vi "Calibration pFC Data.vi"() -> ()   [LabVIEW 2014]
uses:
  <vilib>/Utility/file.llb/Read From Spreadsheet File (DBL).vi
  <vilib>/gmath/NumericalOptimization/Nonlinear Curve Fit LM formula string.vi
  <vilib>/Utility/file.llb/Write To Spreadsheet File (DBL).vi
  <vilib>/Analysis/NI_AALBase.lvlib
  <vilib>/gmath/NI_Gmath.lvlib
  <vilib>/Analysis/NI_AALPro.lvlib
panel:
  out "Selected xDNA (m51 count)":dbl[](array[numeric])
  out "Selected filt xDNA (m51 count)":dbl[](array[numeric])
  out "Selected xDNA (nm)":dbl[](array[numeric])
  in  "Final cut (s)":dbl=120.0
  out "Force (pN)":dbl
  out "read file path":path
  out "Fraction (f-u)":dbl[](array[numeric])
  out "Funfold (%)":dbl
  out "Ffold (%)":dbl
  out "path":path
  in  "Fit?":bool
  in  "initial parameters":dbl[](array[numeric])=[200.0, 1100.0, 6.0, 500.0, 1120.0, 6.0]
  out "Laser Power (mV)":dbl
  out "Data rate (Hz)":dbl
  in  "Tab Control 2":enum32{"Folder", "File"}(tab)
  in  "Folder Path":path
  in  "file path (dialog if empty)":path
  in  "intervals for selected xDNA":i32=100
  out "Histogram: h(x)":i32[](array[numeric])
  out "Selected filt xDNA (nm)":dbl[](array[numeric])
  out "Selected Time (s)":dbl[](array[numeric]) format="%_7g"
  in  "Selected tf (s)":dbl=10.0
  in  "Selected ti (s)":dbl
  out "Time for total (s)":dbl[](array[numeric])
  out "Total Filtered xDNA (nm)":dbl[](array[numeric])
  out "Data rate for total (Hz)":dbl
  in  "Filter for total":T1(ring)=enum."Moving-window avg"
  in  "#Avg for total":i32=5
  in  "# of adjencent points":i32=5
  in  "Save?":bool
  out "Target QPD (V)":dbl
  out "Total xDNA (nm)":dbl[](array[numeric])
  in  "Filter for initial":T1(ring)
  out "Total Peak location (index)":i32[](array[numeric])
  out "Each first and end diff":dbl[](array[numeric])
  out "Total xDNA":dbl[][](array[numeric])
  out "cut-xDNA (nm)":dbl[](array[numeric])
  out "xDNA diff (i-(i+1))":dbl[](array[numeric])
  out "New stage moved index":i32[](array[numeric])
  in  "initial cut (s)":dbl=0.1
  out "Stage moved time index":i32[](array[numeric])
  out "Stage moved time (s)":dbl[](array[numeric])
  out "Time Array (s)":dbl[](array[numeric])
  out "xDNA (nm)":dbl[](array[numeric])
  in  "Tab Control":T2(tab)
  out "XY Graph 4":cluster{dbl[], "Filtered QPD data":dbl[]}[](graph)
  out "XY Graph":cluster{dbl[], dbl[]}(graph)
  out "Each first and end":dbl[](array[numeric])
  out "Each Section First and End index":i32[](array[numeric])
  out "XY Graph 2":cluster{dbl[], dbl[]}(graph)
  out "Waveform Graph":dbl[][](graph)
  out "XY Graph 3":cluster{dbl[], "Filtered QPD data":dbl[]}[](graph)
  out "XY Graph 8":cluster{"power":dbl[], "Slope":dbl[]}(graph)
  out "XY Graph 5":cluster{dbl[], dbl[]}[](graph)
  out "Histogram Graph":T3(graph)
  out "best fit parameters":dbl[](array[numeric])
  out "dx transition (nm)":dbl
  out "XY Graph 7":cluster{dbl[], dbl[]}[](graph)
  in  "3nt binding signal (nm)":dbl=0.5
  out "XY Graph 6":T4(graph)
  out "Spatial Sampling Rate (1/nm)":dbl
  in  "intervals":i32=10
  out "Histogram Graph 2":T5(graph)
  in  "Pairwise?":bool
  out "Upper-Bound QPD radius (nm)":dbl=430.0
  in  "#Avg for initial":i32=25
  out "Data rate for initial (Hz)":dbl
  out "conversion factor (V/um)":dbl=0.75
  in  "Start point of Xbd for pFC (nm)":dbl=300.0
  in  "trap height(nm)":dbl=300.0
  # "try 350 for h=300\n      450 for h=0"
  # "20R xDNA~1100-1120 nm at 13.5 pN\nunfold dx=18 nm"
  # "0.09 for ~290mV"
  # "0.13 for 2800 mV"
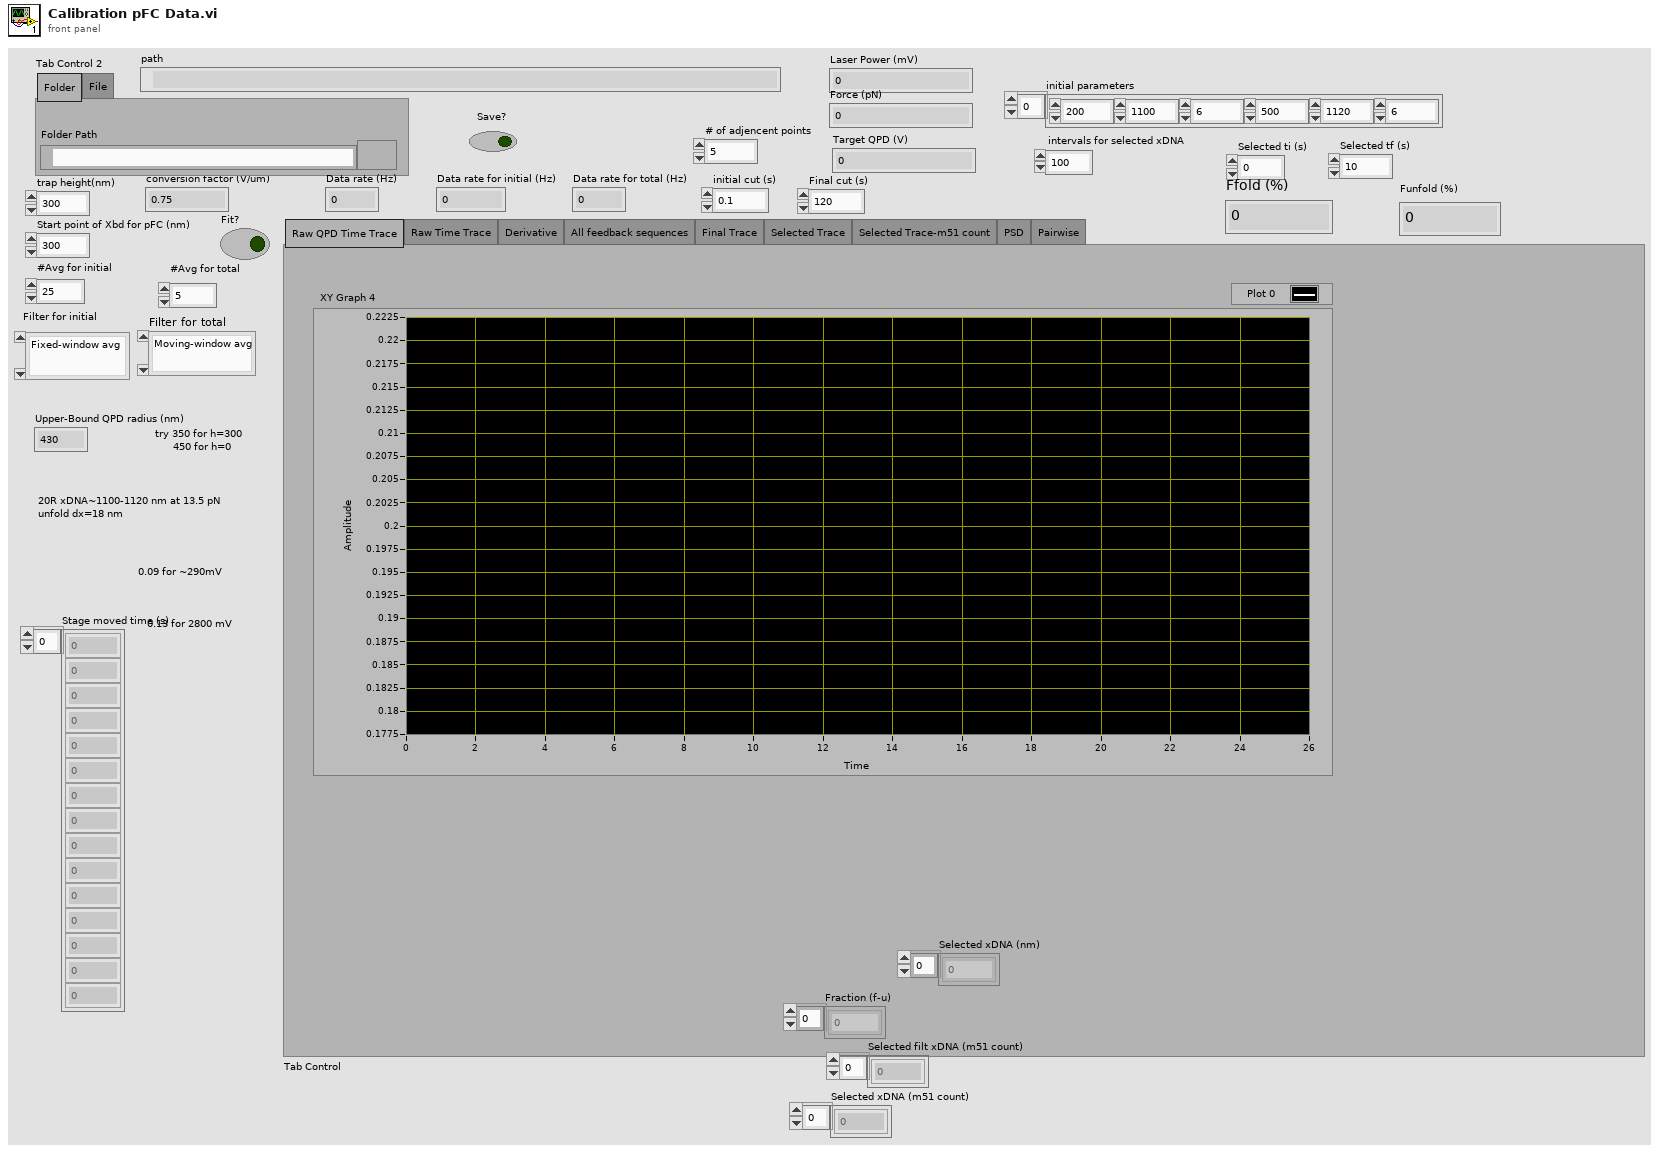
[diagram p1: front panel]
types:
  T1 = enum16{"Fixed-window avg", "Moving-window avg", "F+S-window avg", "S-G filter", "Fixed-window Median", "Moving-window Median "}
  T2 = enum32{"Raw QPD Time Trace", "Raw Time Trace", "Derivative", "All feedback sequences", "Final Trace", "Selected Trace", "Selected Trace-m51 count", "PSD", "Pairwise"}
  T3 = cluster{"X Values":dbl[], "best nonlinear fit":dbl[]}[]
  T4 = cluster{"Frequency (Hz)\n0,df, 2df,...(n/2-1)Fs":dbl[], "Power Spectrum (V^2 rms) (V^2/Hz)":dbl[]}
  T5 = cluster{"X Values":dbl[], "Histogram: h(x)":i32[]}
  T6 = cluster{"model":string, "Parameters":string[], "x":string}
  T7 = cluster{"initial amplitude":dbl, "initial center":dbl, "initial standard deviation":dbl, "offset":dbl}
  T8 = cluster{"X Values":dbl[], "best nonlinear fit":dbl[]}
  T9 = cluster{dbl[], "Power Spectrum (V^2 rms) (V^2/Hz)":dbl[]}
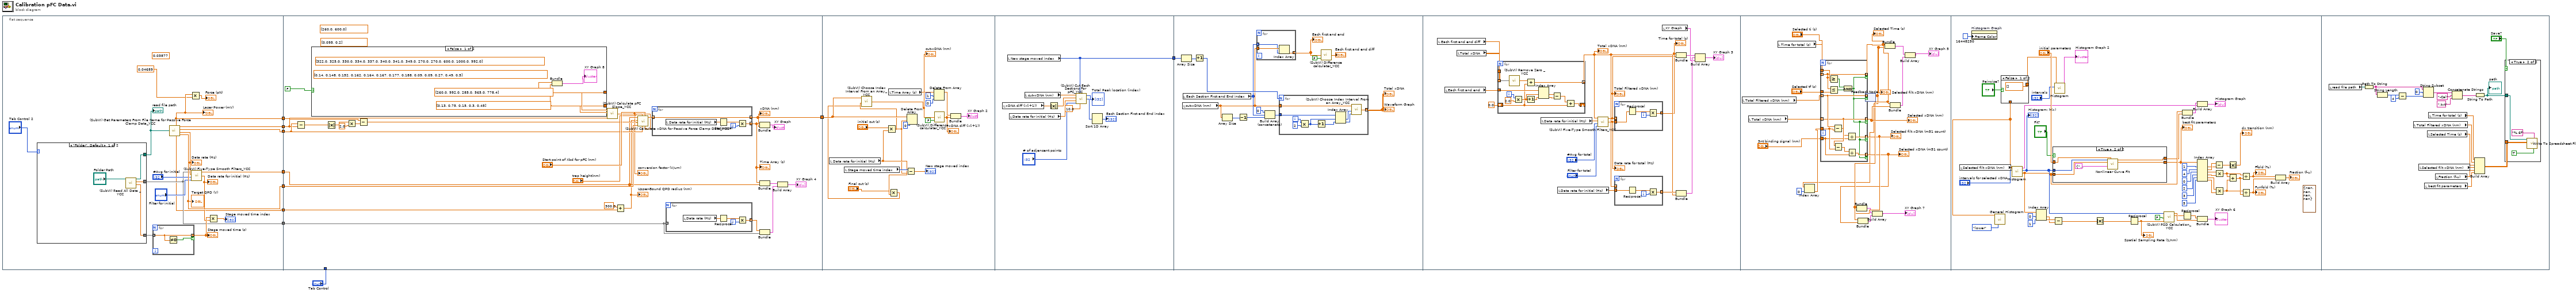
[diagram p0: block diagram]
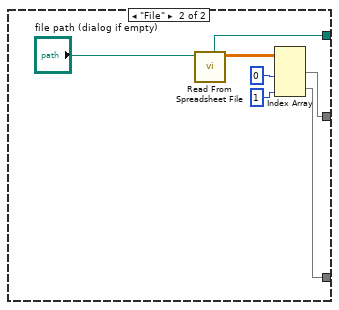
[diagram p2: hidden frame]
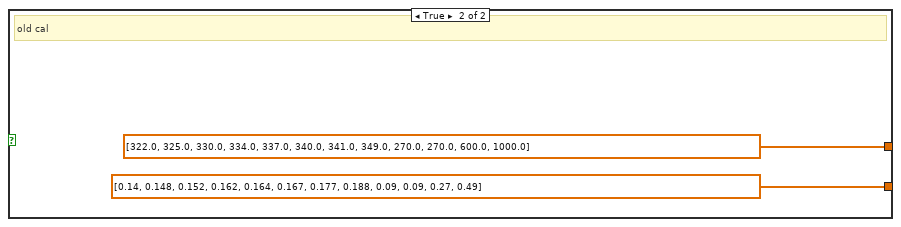
[diagram p3: hidden frame]
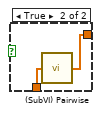
[diagram p4: hidden frame]
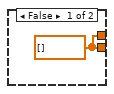
[diagram p5: hidden frame]
diagram:
  n1 = flat-sequence {
    tunnel: [w23] -> w10
    tunnel: [w28] -> w9
    tunnel: [w27] -> w8
    tunnel: [w26] -> w7
    tunnel: [w16] -> w3
    tunnel: [w13] -> w2
    tunnel: [w14] -> w1
    tunnel: "Tab Control" -> [_]
    tunnel: w7 -> [w64]
    tunnel: w8 -> [w65]
    tunnel: w9 -> [w59]
    tunnel: w10 -> [w57]
    tunnel: [w42] -> w5
    tunnel: w3 -> [w52]
    tunnel: w2 -> [w50]
    tunnel: w1 -> [w44]
    tunnel: w5 -> [w89]
    tunnel: [w107] -> w4
    tunnel: w4 -> [w121]
    frame #0 {
      (unwired) 0.03877 ("y")
      n2 = case shown="\"Folder\", Default" "Tab Control 2" {
        tunnel: [w32 w34] -> w18
        tunnel: [w31 w33] -> w17
        tunnel: [w29 w35] -> w16
        frame "Folder", Default {
          n3 = call "(SubVI) Read All Data _YCC.vi"("Folder Path"="Folder Path") -> ("all moved time points"=w32:dbl[], "all QPD data"=w29:dbl[], "Last File Path"=w31:path)  [unwired: 4 in]
        }
        frame "File" {
          n4 = call-poly <vilib>:"Read From Spreadsheet File.vi"("file path (dialog if empty)"="file path (dialog if empty)") -> ("all rows"=w38:dbl[][], "new file path (Not A Path if cancelled)"=w33:path)  [unwired: 6 in, 3 out]
          n5 = Index Array(array=w38, index (col) #1=0 ("disabled index (col)"), index (col) #2=1 ("disabled index (col)")) -> (element #1=w35:dbl[], element #2=w34:dbl[])  [unwired: 2 in]
        }
      }
      "read file path" <- w17
      n6 = for {
        tunnel: [w40] -> w22 mode=indexing if=w41
        tunnel: w18 -> [w40] mode=indexing
        n7 = Not Equal To 0?(x=w40) -> (x != 0?=w41:bool)
      }
      "Stage moved time (s)" <- w22
      n8 = call "(SubVI) Get Paremeters From File Name for Passive Force Clamp Data_YCC.vi"("path"=w17) -> ("Target QPD (V)"=w27:dbl, "Jump (nm)"=w14:dbl, "Data rate (Hz)"=w25:dbl, "Moved position (um)"=w26:dbl, "Laser Power (mV)"=w13:dbl, "Center position (um)"=w28:dbl)  [unwired: 2 in]
      "Target QPD (V)" <- w27
      "Data rate (Hz)" <- w25
      "Laser Power (mV)" <- w13
      n9 = Multiply(x=w13, y=0.04689) -> (x*y=→"Force (pN)":dbl)
      n10 = call "(SubVI) Five-Type Smooth Filters_YCC.vi"("Filter type"="Filter for initial", "Avg points"="#Avg for initial", "Sampling rate (Hz)"=w25, "QPD data"=w16) -> ("Sampling rate after filtering (Hz)"=w21:dbl, "Filtered QPD data"=w23:dbl[])  [unwired: 1 in]
      "Data rate for initial (Hz)" <- w21
      n11 = Multiply(x=w22, y=w21) -> (x*y=→"Stage moved time index":dbl[])
    }
    frame #1 {
      (unwired) dbl[] [0.095, 0.2] ("Slope")
      (unwired) dbl[] [260.0, 600.0] ("power")
      n12 = Subtract(x=w64, y=w59) -> (x-y=w63:dbl)
      n13 = case shown="False" FALSE ("Boolean") {
        tunnel: [w72 dbl[] [322.0, 325.0, 330.0, 334.0, 337.0, 340.0, 341.0, 349.0, 270.0, 270.0, 600.0, 1000.0] ("power")] -> w48
        tunnel: [w71 dbl[] [0.14, 0.148, 0.152, 0.162, 0.164, 0.167, 0.177, 0.188, 0.09, 0.09, 0.27, 0.49] ("Slope")] -> w47
        frame False {
          (unwired) dbl[] [0.14, 0.148, 0.152, 0.162, 0.164, 0.167, 0.177, 0.188, 0.09, 0.09, 0.27, 0.49, 0.5] ("Slope")
          (unwired) dbl[] [322.0, 325.0, 330.0, 334.0, 337.0, 340.0, 341.0, 349.0, 270.0, 270.0, 600.0, 1000.0, 992.0] ("power")
          w71 = dbl[] [0.13, 0.75, 0.15, 0.3, 0.45] ("Slope")
          w72 = dbl[] [260.0, 992.0, 285.0, 565.0, 778.4] ("power")
          n14 = Bundle("power"=w72, "Slope"=w71) -> (→"XY Graph 8":cluster{"power":dbl[], "Slope":dbl[]})  [unwired: 1 in]
        }
        frame True {
          # "old cal"
        }
      }
      n15 = Absolute Value(x=w63) -> (abs(x)=w61:dbl)
      n16 = Multiply(x=w61, y=2.0) -> (x*y=w60:dbl)
      n17 = Subtract(x=w59, y=w60) -> (x-y=w58:dbl)
      n18 = call "(SubVI) Calculate pFC Slope_YCC.vi"("given-power"=w50, "Slope"=w47, "power"=w48) -> ("Cal-slope (V/um)"=w49:dbl)  [unwired: 3 in]
      "conversion factor (V/um)" <- w49
      n19 = Add(x=300.0, y=w44) -> (x+y=w43:dbl)
      "Upper-Bound QPD radius (nm)" <- w43
      n20 = call "(SubVI) Calculate xDNA for Passive Force Clamp Data_YCC.vi"("conversion factor (V/um)"=w49, "Start point of Xbd for pFC (nm)"="Start point of Xbd for pFC (nm)", "Move to (um)"=w64, "trap height(nm)"="trap height(nm)", "QPD center value (V)"=w65, "Stage center point (um)"=w58, "Target QPD radius (nm)"=w43, "QPD Array (V)"=w57) -> ("xDNA (nm)"=w69:dbl[])  [unwired: 1 in, 2 out]
      n21 = for {
        tunnel: w69 -> [w79] mode=indexing
        tunnel: [w80] -> w56 mode=indexing
        tunnel: [w79] -> w42 mode=indexing
        i -> [w83]
        n22 = local read "Data rate for initial (Hz)"() -> (w82:dbl)
        n23 = Reciprocal(x=w82) -> (1/x=w81:dbl)
        n24 = Multiply(x=w81, y=w83) -> (x*y=w80:dbl)
      }
      "xDNA (nm)" <- w42
      "Time Array (s)" <- w56
      n25 = for {
        tunnel: w52 -> [_] mode=indexing
        tunnel: [w75] -> w51 mode=indexing
        i -> [w76]
        n26 = local read "Data rate (Hz)"() -> (w78:dbl)
        n27 = Reciprocal(x=w78) -> (1/x=w77:dbl)
        n28 = Multiply(x=w77, y=w76) -> (x*y=w75:dbl)
      }
      n29 = Bundle(w56, w42) -> (→"XY Graph":cluster{dbl[], dbl[]})  [unwired: 1 in]
      n30 = Bundle(w56, "Filtered QPD data"=w57) -> (w53:cluster{dbl[], "Filtered QPD data":dbl[]})  [unwired: 1 in]
      n31 = Bundle(w51, "all rows"=w52) -> (w54:cluster{dbl[], "all rows":dbl[]})  [unwired: 1 in]
      n32 = Build Array(w53, w54) -> (→"XY Graph 4":cluster{dbl[], "all rows":dbl[]}[])
    }
    frame #2 {
      n33 = local read "Data rate for initial (Hz)"() -> (w88:dbl)
      n34 = local read "Stage moved time index"() -> (w91:i32[])
      n35 = Multiply(x="initial cut (s)", y=w88) -> (x*y=w86:dbl)
      n36 = local read "Time Array (s)"() -> (w100:dbl[])
      n37 = Multiply(x="Final cut (s)", y=w88) -> (x*y=w85:dbl)
      n38 = call "(SubVI) Choose Index Interval From an Array_YCC.vi"("End index"=w85, "Start index"=w86, "array"=w89) -> ("Array out"=w84:dbl[])  [unwired: 3 in]
      "cut-xDNA (nm)" <- w84
      n39 = Subtract(x=w91, y=w86) -> (x-y=→"New stage moved index":dbl[])
      n40 = Delete From Array(array=w89, length=w86, index=0) -> ()  [unwired: 2 out]
      n41 = Delete From Array(array=w100, length=1, index=0) -> (array with subset deleted=w96:dbl[])  [unwired: 1 out]
      n42 = call "(SubVI) Difference calculater_YCC.vi"("T= (i+1)-i\nF=i-(i+1)"=FALSE ("T= (i+1)-i\nF=i-(i+1)"), "Array in"=w84) -> ("Diff"=w95:dbl[])  [unwired: 3 in]
      "xDNA diff (i-(i+1))" <- w95
      n43 = Bundle("Time Array (s)"=w96, "Diff"=w95) -> (→"XY Graph 2":cluster{"Time Array (s)":dbl[], "Diff":dbl[]})  [unwired: 1 in]
    }
    frame #3 {
      n44 = local read "xDNA diff (i-(i+1))"() -> (w104:dbl[])
      n45 = local read "New stage moved index"() -> (w107:i32[])
      n46 = local read "Data rate for initial (Hz)"() -> (w108:dbl)
      n47 = local read "cut-xDNA (nm)"() -> (w109:dbl[])
      n48 = Absolute Value(x=w104) -> (abs(x)=w103:dbl[])
      n49 = call "(SubVI) Cut Each Sections For pFC_YCC.vi"("xDNA"=w109, "Initial guess locations"=w107, "Diff (i-i+1)"=w103, "Data Rate (Hz)"=w108, "threshold y"=10.0, "# of adjencent points"="# of adjencent points") -> ("Total Peak location (index)"=→"Total Peak location (index)":i32[], "Each Section First and End index"=w102:i32[])  [unwired: 1 in]
      n50 = Sort 1D Array(array=w102) -> (sorted array=→"Each Section First and End index":i32[])
    }
    frame #4 {
      n51 = Array Size(array=w121) -> (size(s)=w120:i32)
      n52 = local read "cut-xDNA (nm)"() -> (w112:dbl[])
      n53 = local read "Each Section First and End index"() -> (w113:i32[])
      n54 = Increment(x=w120) -> (x+1=w119:i32)
      n55 = Array Size(array=w112) -> (size(s)=w116:i32)
      n56 = Decrement(x=w116) -> (x-1=w115:i32)
      n57 = for {
        tunnel: w113 -> [w125] mode=indexing
        tunnel: w112 -> [w126]
        tunnel: [w124] -> w111 mode=indexing
        n58 = Index Array(array=w126, index=w125) -> (element=w124:dbl)
      }
      "Each first and end" <- w111
      n59 = Build Array (concatenate)(0, w113, w115) -> (w117:i32[])
      n60 = for {
        N: w119 -> [_]
        tunnel: w112 -> [w135]
        tunnel: w117 -> [w134]
        tunnel: [w128] -> w114 mode=indexing
        i -> [w127]
        n61 = Multiply(x=w127, y=2) -> (x*y=w130:i32)
        n62 = Increment(x=w130) -> (x+1=w129:i32)
        n63 = Index Array(array=w134, index #1=w130, index #2=w129) -> (element #1=w133:i32, element #2=w132:i32)
        n64 = call "(SubVI) Choose Index Interval From an Array_YCC.vi"("End index"=w132, "Start index"=w133, "array"=w135) -> ("Array out"=w128:dbl[])  [unwired: 3 in]
      }
      "Waveform Graph" <- w114
      "Total xDNA" <- w114
      n65 = call "(SubVI) Difference calculater_YCC.vi"("T= (i+1)-i\nF=i-(i+1)"=FALSE ("T= (i+1)-i\nF=i-(i+1)"), "Array in"=w111) -> ("Diff"=→"Each first and end diff":dbl[])  [unwired: 3 in]
    }
    frame #5 {
      n66 = local read "Each first and end diff"() -> (w152:dbl[])
      n67 = local read "Each first and end"() -> (w151:dbl[])
      n68 = local read "Total xDNA"() -> (w147:dbl[][])
      n69 = for {
        tunnel: w147 -> [w172] mode=indexing
        tunnel: w152 -> [_]
        tunnel: [w173] -> w146 mode=concatenating
        tunnel: w151 -> [w166]
        shift-right: [w162] -> _
        shift-left: 0.0 -> [w161]
        i -> [w169]
        n70 = call "(SubVI) Remove Zero _YCC.vi"("Array in"=w172) -> ("Array out"=w171:dbl[])  [unwired: 4 in]
        n71 = Multiply(x=w169, y=2.0) -> (x*y=w168:dbl)
        n72 = Add(x=w171, y=w161) -> (x+y=w173:dbl[])
        n73 = Increment(x=w168) -> (x+1=w167:dbl)
        n74 = Index Array(array=w166, index #1=w168, index #2=w167) -> (element #1=w165:dbl, element #2=w164:dbl)
        n75 = Subtract(x=w165, y=w164) -> (x-y=w163:dbl)
        n76 = Add(x=w163, y=w161) -> (x+y=w162:dbl)
      }
      "Total xDNA (nm)" <- w146
      n77 = local read "Data rate for initial (Hz)"() -> (w145:dbl)
      n78 = local read "Data rate for initial (Hz)"() -> (w149:dbl)
      n79 = call "(SubVI) Five-Type Smooth Filters_YCC.vi"("Filter type"="Filter for total", "Avg points"="#Avg for total", "Sampling rate (Hz)"=w145, "QPD data"=w146) -> ("Sampling rate after filtering (Hz)"=w139:dbl, "Filtered QPD data"=w140:dbl[])  [unwired: 1 in]
      "Data rate for total (Hz)" <- w139
      "Total Filtered xDNA (nm)" <- w140
      n80 = for {
        tunnel: w139 -> [w156]
        tunnel: [w154] -> w138 mode=indexing
        tunnel: w140 -> [_] mode=indexing
        i -> [w153]
        n81 = Reciprocal(x=w156) -> (1/x=w155:dbl)
        n82 = Multiply(x=w155, y=w153) -> (x*y=w154:dbl)
      }
      "Time for total (s)" <- w138
      n83 = for {
        tunnel: w146 -> [_] mode=indexing
        tunnel: w149 -> [w160]
        tunnel: [w158] -> w148 mode=indexing
        i -> [w157]
        n84 = Reciprocal(x=w160) -> (1/x=w159:dbl)
        n85 = Multiply(x=w159, y=w157) -> (x*y=w158:dbl)
      }
      n86 = local read "XY Graph"() -> (w136:cluster{dbl[], dbl[]})
      n87 = Bundle(w138, "Filtered QPD data"=w140) -> (w141:cluster{dbl[], "Filtered QPD data":dbl[]})  [unwired: 1 in]
      n88 = Bundle(w148, w146) -> (w142:cluster{dbl[], dbl[]})  [unwired: 1 in]
      n89 = Build Array(w141, w142, w136) -> (→"XY Graph 3":cluster{dbl[], "Filtered QPD data":dbl[]}[])
    }
    frame #6 {
      n90 = local read "Total Filtered xDNA (nm)"() -> (w185:dbl[])
      n91 = local read "Total xDNA (nm)"() -> (w190:dbl[])
      n92 = local read "Time for total (s)"() -> (w193:dbl[])
      n93 = feedback #1() -> (w174:dbl[])  [unwired: 1 in]
      "Selected filt xDNA (nm)" <- w174
      n94 = Index Array(array=w174, index=0) -> (element=w183:dbl)
      n95 = for {
        tunnel: w193 -> [w206] mode=indexing
        tunnel: [w202] -> w175 mode=indexing if=w194
        tunnel: w185 -> [w202] mode=indexing
        tunnel: [w206] -> w181 mode=indexing if=w194
        tunnel: "Selected ti (s)" -> [w207]
        tunnel: "Selected tf (s)" -> [w205]
        tunnel: w190 -> [w201] mode=indexing
        tunnel: [w201] -> w189 mode=indexing if=w194
        tunnel: w183 -> [w200]
        tunnel: "3nt binding signal (nm)" -> [w197]
        tunnel: [w196] -> w180 mode=indexing if=w194
        tunnel: [w195] -> w178 mode=indexing if=w194
        n96 = Greater Or Equal?(x=w206, y=w207) -> (x >= y?=w204:bool)
        n97 = Less Or Equal?(x=w206, y=w205) -> (x <= y?=w203:bool)
        n98 = Subtract(x=w202, y=w200) -> (x-y=w199:dbl)
        n99 = Subtract(x=w201, y=w200) -> (x-y=w198:dbl)
        n100 = And(x=w204, y=w203) -> (x .and. y?=w194:bool)
        n101 = Divide(x=w199, y=w197) -> (x/y=w196:dbl)
        n102 = Divide(x=w198, y=w197) -> (x/y=w195:dbl)
      }
      "Selected Time (s)" <- w181
      "Selected xDNA (nm)" <- w189
      "Selected filt xDNA (m51 count)" <- w180
      "Selected xDNA (m51 count)" <- w178
      n103 = Bundle(w181, w180) -> (w179:cluster{dbl[], dbl[]})  [unwired: 1 in]
      n104 = Bundle(w181, w178) -> (w177:cluster{dbl[], dbl[]})  [unwired: 1 in]
      n105 = feedback-in #1(w175) -> ()
      n106 = Build Array(w179, w177) -> (→"XY Graph 7":cluster{dbl[], dbl[]}[])
      n107 = Bundle(w181, w174) -> (w187:cluster{dbl[], dbl[]})  [unwired: 1 in]
      n108 = Bundle(w181, w189) -> (w186:cluster{dbl[], dbl[]})  [unwired: 1 in]
      n109 = Build Array(w187, w186) -> (→"XY Graph 5":cluster{dbl[], dbl[]}[])
    }
    frame #7 {
      (unwired) T7 {"initial amplitude"=nan, "initial center"=nan, "initial standard deviation"=nan, "offset"=nan} ("initial guess")
      n110 = local read "Selected filt xDNA (nm)"() -> (w209:dbl[])
      n111 = property on="Histogram Graph" class="XYGraph (strict)"("Frame Color"=u32 16448250) -> ()  [unwired: 2 in, 2 out]
      n112 = call <vilib>:"General Histogram.vi"("X"=w209, "inclusion"=enum32{"lower", "upper"}."lower") -> ()  [unwired: 9 in, 5 out]
      n113 = case shown="False" "Pairwise?" {
        tunnel: w209 -> [_ w259]
        tunnel: [dbl[] [] ("Pairwise") w258] -> w213
        frame False {
        }
        frame True {
          n114 = call "(SubVI) Pairwise.vi"("Data"=w259) -> ("Pairwise"=w258:dbl[])  [unwired: 4 in]
        }
      }
      n115 = call <vilib>:"Histogram.vi"("intervals"="intervals for selected xDNA", "X"=w209) -> ("X Values"=w243:dbl[], "Histogram: h(x)"=w245:i32[], "Histogram Graph"=w240:T5)  [unwired: 6 in, 1 out]
      "Histogram: h(x)" <- w245
      n116 = Index Array(array=w243, index #1=0 ("index"), index #2=1 ("index")) -> (element #1=w251:dbl, element #2=w252:dbl)
      n117 = case shown="True" "Fit?" {
        tunnel: w245 -> [_ w265]
        tunnel: "initial parameters" -> [_ w264]
        tunnel: w243 -> [_ w263]
        tunnel: [w260 w262] -> w242
        tunnel: [w260 w261] -> w238
        frame False {
          w260 = dbl[] [] ("best nonlinear fit")
        }
        frame True {
          n118 = call-poly <vilib>:"Nonlinear Curve Fit.vi"("Y"=w265, "initial parameters"=w264, "X"=w263, "model description"=T6 {"model"="a1*exp(-((u-a2)/a3)^2)+a4*exp(-((u-a5)/a6)^2)", "Parameters"=["a1", "a2", "a3", "a4", "a5", "a6"], "x"="u"}) -> ("best nonlinear fit"=w262:dbl[], "best fit parameters"=w261:dbl[])  [unwired: 7 in, 3 out]
        }
      }
      "best fit parameters" <- w238
      n119 = Subtract(x=w252, y=w251) -> (x-y=w250:dbl)
      n120 = call <vilib>:"Histogram.vi"("intervals"="intervals", "X"=w213) -> ("Histogram Graph"=→"Histogram Graph 2":T5)  [unwired: 6 in, 3 out]
      n121 = Absolute Value(x=w250) -> (abs(x)=w249:dbl)
      n122 = Reciprocal(x=w249) -> (1/x=w248:dbl)
      "Spatial Sampling Rate (1/nm)" <- w248
      n123 = call "(SubVI) PSD Calculation_YCC.vi"("sampling frequency (Hz)"=w248, "T=NI made PSD\nF=YCC made PSD"=FALSE ("T=NI made PSD\nF=YCC made PSD"), "QPD data"=w245) -> ("Frequency (Hz)\n0,df, 2df,...(n/2-1)Fs"=w230:dbl[], "Power Spectrum (V^2 rms) (V^2/Hz)"=w247:dbl[])  [unwired: 3 in]
      n124 = Reciprocal(x=w230) -> (1/x=w229:dbl[])
      n125 = Bundle("X Values"=w243, "best nonlinear fit"=w242) -> (w239:T8)  [unwired: 1 in]
      n126 = Index Array(array=w238, index #1=1 ("index"), index #2=4 ("index"), index #3=0 ("index"), index #4=2 ("index"), index #5=3 ("index"), index #6=5 ("index")) -> (element #1=w234:dbl, element #2=w235:dbl, element #3=w224:dbl, element #4=w223:dbl, element #5=w222:dbl, element #6=w221:dbl)
      n127 = Build Array(w239, w240) -> (→"Histogram Graph":T3)
      n128 = Bundle(w229, "Power Spectrum (V^2 rms) (V^2/Hz)"=w247) -> (→"XY Graph 6":T9)  [unwired: 1 in]
      n129 = Subtract(x=w235, y=w234) -> (x-y=w233:dbl)
      n130 = Multiply(x=w224, y=w223) -> (x*y=w220:dbl)
      n131 = Multiply(x=w222, y=w221) -> (x*y=w218:dbl)
      n132 = Absolute Value(x=w233) -> (abs(x)=→"dx transition (nm)":dbl)
      n133 = Add(x=w220, y=w218) -> (x+y=w219:dbl)
      n134 = Divide(x=w220, y=w219) -> (x/y=w217:dbl)
      "Ffold (%)" <- w217
      n135 = Divide(x=w218, y=w219) -> (x/y=w216:dbl)
      "Funfold (%)" <- w216
      n136 = Build Array(w217, w216) -> (→"Fraction (f-u)":dbl[])
    }
    frame #8 {
      n137 = local read "read file path"() -> (w279:path)
      n138 = Path To String(path=w279) -> (string=w274:string)
      n139 = String Length(string=w274) -> (length=w278:i32)
      n140 = Subtract(x=w278, y=4) -> (x-y=w276:i32)
      n141 = local read "Total Filtered xDNA (nm)"() -> (w283:dbl[])
      n142 = local read "Selected filt xDNA (nm)"() -> (w281:dbl[])
      n143 = String Subset(string=w274, offset (0)=0, length (rest)=w276) -> (substring=w273:string)
      n144 = local read "best fit parameters"() -> (w267:dbl[])
      n145 = local read "Selected Time (s)"() -> (w280:dbl[])
      n146 = local read "Time for total (s)"() -> (w284:dbl[])
      n147 = local read "Fraction (f-u)"() -> (w268:dbl[])
      n148 = Concatenate Strings(w273, "-Cal" ("string"), ".txt" ("string")) -> (w270:string)
      n149 = String To Path(string=w270) -> (path=w269:path)
      "path" <- w269
      n150 = Build Array(w284, w283, w280, w281, w268, w267) -> (w282:dbl[][])
      n151 = case shown="True" "Save?" {
        tunnel: w282 -> [_ w287]
        tunnel: w269 -> [_ w286]
        frame False {
        }
        frame True {
          n152 = call-poly <vilib>:"Write To Spreadsheet File.vi"("transpose? (no:F)"=TRUE, "format (%.3f)"="%.6f", "2D data"=w287, "file path (dialog if empty)"=w286) -> ()  [unwired: 4 in, 1 out]
        }
      }
    }
  }
